vi "Unclassified_2222.vi"   [LabVIEW 2015]
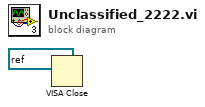
[diagram p0: block diagram]
diagram:
  n1 = VISA Close(VISA resource name=refnum<visa-resource-name> "COM3" ("VISA资源名称")) -> ()  [unwired: 1 in, 1 out]
